vi "RestartSequenceAcquistion.vi"(8 "error in (no error)":errorcluster, 11 "Camera_Prime95B in":refnum<class "Camera_Prime95B.lvclass">) -> (0 "error out":errorcluster, 3 "Camera_Prime95B out":refnum<class "Camera_Prime95B.lvclass">)   [LabVIEW 2020, in "Camera_Prime95B.lvlib" / "Camera_Prime95B.lvclass"]
uses:
  Camera_Prime95B.lvclass
  Hardware Abstraction Layer/Component/Device/Device/DataExchange.ctl
  Camera_Prime95B.lvclass/Camera_Prime95B.ctl
  Interface/DataListener/DataListener.lvclass
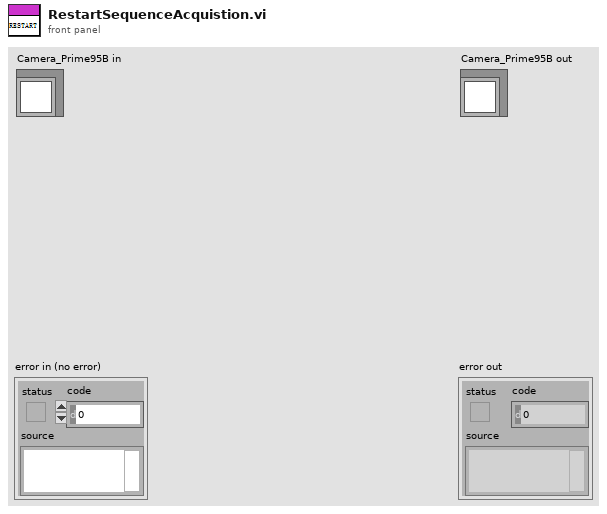
[diagram p1: front panel]
types:
  T1 = typedef "DataListener.lvclass/DataExchange.ctl" = cluster{"Source":string, "Target":string, "Type":string, "value":variant}
  T2 = typedef "Camera_Prime95B.lvlib/Camera_Prime95B.lvclass/AcquisitionParams.ctl" = cluster{"ExposureMs":dbl, "Frames":dbl, "Interval":dbl, "Save Path":path, "Stream Save Path":path, "SingleStack?":bool, "StreamToDisk?":bool, "Alert when finish?":bool, "File suffix":string, "Live?":bool}
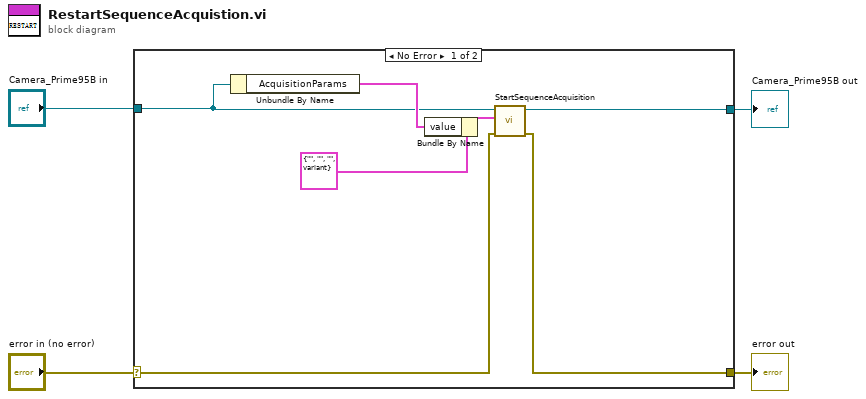
[diagram p0: block diagram]
diagram:
  n1 = case shown="No Error" "error in (no error)" {
    selector: "error in (no error)" -> [w6 w13]
    tunnel: [w5 w13] -> w3
    tunnel: [w7 w12] -> w1
    tunnel: "Camera_Prime95B in" -> [w8 w12]
    frame No Error {
      n2 = Unbundle By Name(w8) -> ("AcquisitionParams"=w9:T2)
      n3 = Bundle By Name(cluster=T1 {"Source"="", "Target"="", "Type"="", "value"=variant} ("DataExchange"), "value"=w9) -> (w10:T1)
      n4 = call-dynamic "StartSequenceAcquisition.vi"("error in (no error)"=w6, "DataExchange"=w10, "Camera_Prime95B in"=w8) -> ("error out"=w5:errorcluster, "Camera_Prime95B out"=w7:refnum<class "Camera_Prime95B.lvclass">)  [unwired: 7 in]
    }
    frame Error {
    }
  }
  "error out" <- w3
  "Camera_Prime95B out" <- w1
